vi "MRC Allocate String.vi"(8 "error in (no error)":errorcluster, 10 "length":i64, 11 "mrcString":cluster{"str":u64, "len":i64}) -> (0 "error out":errorcluster, 1 "function return":string, 2 "str":string, 3 "mrcString out":cluster{"str":u64, "len":i64})   [LabVIEW 2026, in "MrcLib.lvlib"]
doc: "char* MRC_CALLCONV MRC_AllocateString(struct MRC_String* mrcString, size_t length);"
uses:
  MrcLib.lvlib
  MrcLib.dll
  <vilib>/Utility/importsl/GetValueByPointer/GetValueByPointer.xnode
  <vilib>/Utility/importsl/GetValueByPointer/datatype.ctl
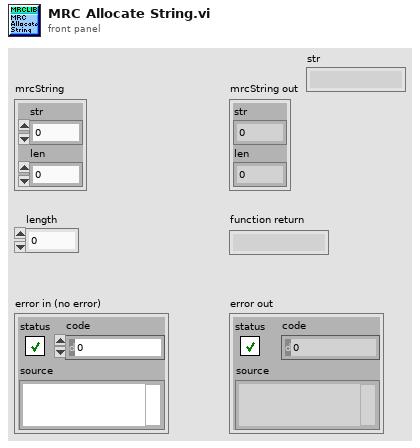
[diagram p1: front panel]
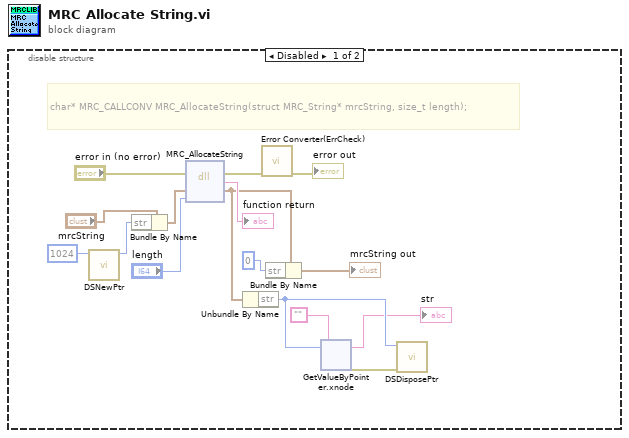
[diagram p0: block diagram]
diagram:
  n1 = disable-structure shown="Disabled" {
    frame Disabled {
      # "char* MRC_CALLCONV MRC_AllocateString(struct MRC_String* mrcString, size_t length);"
      n2 = call <vilib>:"DSNewPtr.vi"("Size"=u64 1024) -> ("Pointer"=w13:u64)  [unwired: 9 in, 1 out]
      n3 = Bundle By Name(cluster="mrcString", "str"=w13) -> (w12:cluster{"str":u64, "len":i64})
      n4 = dll-call lib="MrcLib.*" fn="MRC_AllocateString"(error in="error in (no error)", "mrcString"=w12, "length"="length") -> (error out=w2:errorcluster, →"function return":string, "mrcString"=w7:cluster{"str":u64, "len":i64})  [unwired: 3 in, 1 out]
      n5 = Unbundle By Name(w7) -> ("str"=w10:u64)
      n6 = call <vilib>:"Error Converter(ErrCheck).vi"("error in (no error)"=w2) -> ("error out"=→"error out":errorcluster)  [unwired: 10 in]
      n7 = Bundle By Name(cluster=w7, "str"=u64 0) -> (→"mrcString out":cluster{"str":u64, "len":i64})
      n8 = xnode "GetValueByPointer.xnode"("Pointer"=w10, "InputType"="") -> ("Output"=→"str":string, "ErrorOut"=w11:errorcluster)  [unwired: 2 in]
      n9 = call <vilib>:"DSDisposePtr.vi"("error in (no error)"=w11, "Pointer"=w10) -> ()  [unwired: 9 in, 1 out]
    }
    frame Enabled {
    }
  }
